vi "combine vectors.vi"(9 "magnitudes":sgl[](array[numeric]), 11 "directions":sgl[](array[numeric])) -> (1 "magnitude":sgl, 3 "direction":sgl)   [LabVIEW 2009]
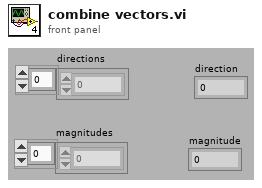
[diagram p1: front panel]
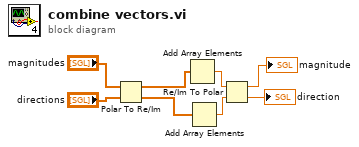
[diagram p0: block diagram]
diagram:
  n1 = Polar To Re/Im(2:"directions", 3:"magnitudes") -> (0:w7:sgl[], 1:w8:sgl[])
  n2 = Add Array Elements(numeric array=w8) -> (sum=w5:sgl)
  n3 = Add Array Elements(numeric array=w7) -> (sum=w6:sgl)
  n4 = Re/Im To Polar(2:w6, 3:w5) -> (0:→"direction":sgl, 1:→"magnitude":sgl)
